vi "Service Location FGV.vi"(8 "error in":errorcluster, 9 "location unique id in":u64, 10 "resolve service request":T2, 11 "action":T1) -> (0 "error out":errorcluster, 1 "location unique id out":u64, 3 "service location":T3)   [LabVIEW 2020, in "Plug-In SDK Discovery V1 API.lvlib"]
uses:
  Plug-In SDK Discovery V1 API.lvlib
  Resolve Service.vi
  gRPC/Generated APIs/ni/measurementlink/discovery/v1/RPC Messages/ni_measurementlink_discovery_v1_ServiceLocation.ctl
  gRPC/Generated APIs/ni/measurementlink/discovery/v1/ni.measurementlink.discovery.v1.lvlib
  gRPC/Generated APIs/ni/measurementlink/discovery/v1/RPC Messages/ni_measurementlink_discovery_v1_ResolveServiceRequest.ctl
  TypeDefs/Service Location FGV Action.ctl
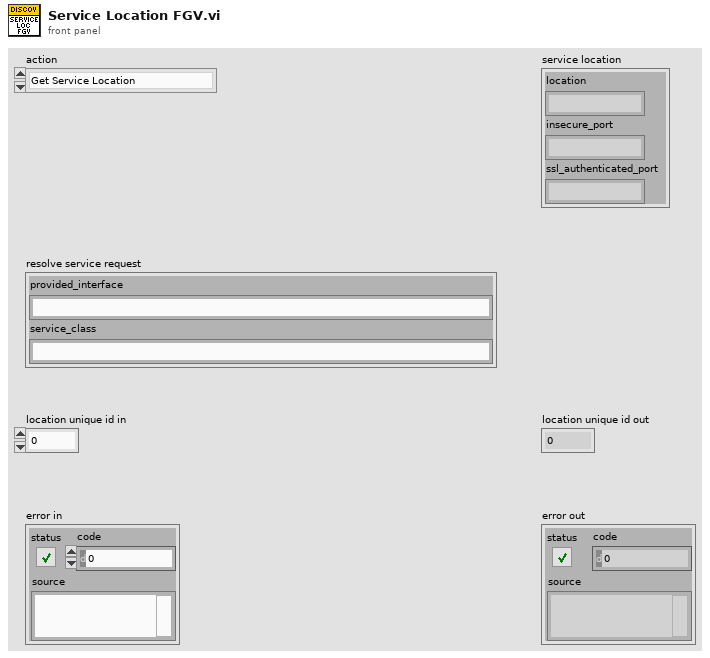
[diagram p1: front panel]
types:
  T1 = typedef "Plug-In SDK Discovery V1 API.lvlib/Service Location FGV Action.ctl" = enum16{"Get Service Location", "Reresolve Service Location"}
  T2 = typedef "ni.measurementlink.discovery.v1.lvlib/ni_measurementlink_discovery_v1_ResolveServiceRequest.ctl" = cluster{"provided_interface":string, "service_class":string}
  T3 = typedef "ni.measurementlink.discovery.v1.lvlib/ni_measurementlink_discovery_v1_ServiceLocation.ctl" = cluster{"location":string, "insecure_port":string, "ssl_authenticated_port":string}
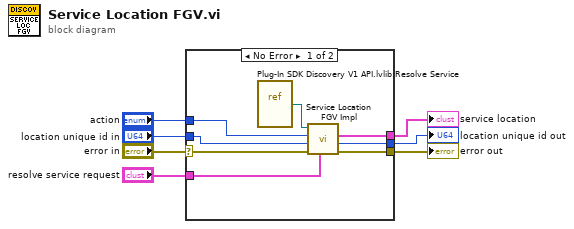
[diagram p0: block diagram]
diagram:
  n1 = case shown="No Error" "error in" {
    selector: "error in" -> [w11 w16]
    tunnel: [w10 w16] -> w5
    tunnel: [w9 _] -> w7
    tunnel: "resolve service request" -> [w12 _]
    tunnel: "action" -> [w14 _]
    tunnel: [w8 _] -> w2
    tunnel: "location unique id in" -> [w13 _]
    frame No Error {
      n2 = vi-ref "Plug-In SDK Discovery V1 API.lvlib:Resolve Service.vi"() -> (w15:refnum<vi>)
      n3 = call "Service Location FGV Impl.vi"("resolve service request"=w12, "error in"=w11, "location unique id in"=w13, "action"=w14, "resolve vi reference"=w15) -> ("error out"=w10:errorcluster, "location unique id out"=w8:u64, "service location"=w9:T3)  [unwired: 4 in]
    }
    frame Error {
    }
  }
  "service location" <- w7
  "error out" <- w5
  "location unique id out" <- w2
